vi "Read_bin_send_to_text.vi"(8 "error in (no error)":errorcluster, 11 "Byte Stream File in":refnum<file>) -> (0 "error out":errorcluster)   [LabVIEW 2017, in "labview-standard-library.lvlib"]
uses:
  labview-standard-library.lvlib
  Event_log_binary_data.ctl
  Time&Event_cluster.ctl
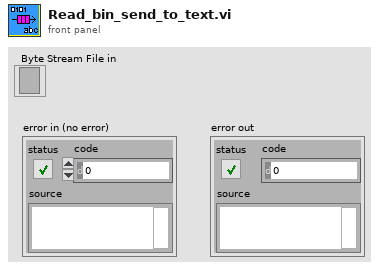
[diagram p1: front panel]
types:
  T1 = typedef "labview-standard-library.lvlib/Time&Event_cluster.ctl" = cluster{"Time in seconds":dbl, "Event text":string}
  T2 = typedef "labview-standard-library.lvlib/Event_log_binary_data.ctl" = cluster{"path":path, "Time/Event":T1[]}
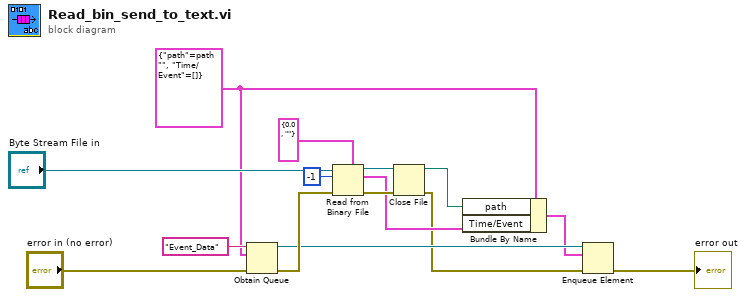
[diagram p0: block diagram]
diagram:
  w6 = T2 {"path"=path "", "Time/Event"=[]}
  n1 = Obtain Queue(name (unnamed)="Event_Data", element data type=w6, error in (no error)="error in (no error)") -> (queue out=w8:refnum<queue>, error out=w9:errorcluster)  [unwired: 2 in, 1 out]
  n2 = Read from Binary File(5:T1 {"Time in seconds"=0.0, "Event text"=""} ("element 2"), 8:w9, 10:-1 ("count (1)"), 11:"Byte Stream File in") -> (0:w11:errorcluster, 2:w3:T1[], 3:w12:refnum<file>)  [unwired: 2 in, 1 out]
  n3 = Close File(refnum=w12, error in=w11) -> (path=w5:path, error out=w2:errorcluster)
  n4 = Bundle By Name(cluster=w6, "path"=w5, "Time/Event"=w3) -> (w7:T2)
  n5 = Enqueue Element(queue=w8, element=w7, error in (no error)=w2) -> (error out=→"error out":errorcluster)  [unwired: 1 in, 2 out]
